vi "20220818_Etalon_with_peak_tracking_for_beam_deviation_working2 .vi"(0 "Session In":T3) -> (4 "vrt. slope":dbl format="%#_9g", 6 "vert intercept":dbl)   [LabVIEW 2021]
uses:
  <vilib>/userDefined/High Color/IMAQdx.ctl
  <vilib>/Analysis/2dsp.llb/Integral Method.ctl
  <vilib>/Analysis/coordinate.llb/2D Cartesian Coordinate Rotation (Array).vi
  <vilib>/Analysis/8numeric.llb/1D Numeric Integration.vi
  <vilib>/Analysis/6fits.llb/Confidence Interval (Linear).vi
  <vilib>/Instr/_visa.llb/VISA Configure Serial Port (Instr).vi
  <vilib>/addons/control/pid/pid.llb/PID (DBL).vi
  <vilib>/Analysis/3filter.llb/Butterworth Filter (DBL).vi
  <vilib>/vision/driver/NI_Vision_Acquisition_Software.lvlib
  <vilib>/Analysis/NI_AALPro.lvlib
  <vilib>/Analysis/NI_AALBase.lvlib
  <vilib>/Analysis/NI_AAL_SigProc.lvlib
  <vilib>/ptbypt/NI_PtbyPt.lvlib
  <resource>/objmgr/imaqdx.rc
  <vilib>/addons/control/pid/NI_PID_pid.lvlib
panel:
  out "second pass wl":dbl format="%#_9g"
  in  "wedge angle (rad)":dbl=0.008737255226 format="%#_13g"
  in  "wedge spacing":dbl=0.8629192 step=1e-06 format="%#_13g"
  in  "pixel size (nm)":dbl=4500.0 format="%#_13g"
  in  "window 2":dbl
  in  "window 1":dbl
  out "Verticle slope (distance between two consecutive fringes)":cluster{dbl[], dbl[]}(graph)
  out "vertical Fringes":dbl[](graph)
  out "Vertical intercept vs real time":cluster{dbl[], dbl[]}(graph)
  out "process variable":dbl
  in  "second peak":i32
  out "Waveform Graph":dbl[](graph)
  out "result 2":dbl format="%0.4f"
  out "Area":dbl
  out "result":dbl format="%0.4f"
  out "First peak pos":dbl
  in  "First peak":i32
  in  "end":dbl format="%.2f"
  in  "index":i32=10
  in  "length":i32=960
  in  "index 2":i32=30
  in  "length 2":i32=700
  out "horzontal intercept":cluster{dbl[], dbl[]}(graph)
  out "horz intercept value":dbl[](array[numeric])
  out "vert wavelength":cluster{dbl[], dbl[]}(graph)
  out "intercept":dbl
  out "x/y":dbl[][](array[numeric])
  out "vert.wl":dbl
  out "d value":dbl format="%#_10e"
  in  "contrast":ext(slide)=0.16666666666666666 scale=0.0..0.3 scale format="%#_12g"
  in  "order 2":i32=2
  in  "order":i32=2
  in  "thor wedge spacing":dbl=4.997771500000001 step=1e-06 format="%#_13g"
  in  "wedge angle of thor wedge":dbl=0.004681980000000043 format="%#_13g"
  in  "horz. fringe width":i32=6 min=3
  out "hor. std dev":dbl format="%0.5f"
  in  "camera property":bool
  in  "saturation":u32(slide) scale=0.0..128.0
  in  "Gain":u32(slide)=49 scale=1.0..256.0
  in  "exposure":ext(slide)=0.49047851562500955 scale=0.000122070313..1.0 scale format="%#_12g"
  out "EnumStrings[]":string[](array[string])
  in  "Numeric":dbl
  out "known wavelength":dbl
  in  "vert width":i32=3 min=3
  out "vert loc":dbl[](array[numeric])
  out "Locations":dbl[](array[numeric])
  out "x > y?":bool
  out "Buffer Number Out":u32
  out "observed wavelength":dbl
  out "horz.intercept":dbl format="%#_8g"
  out "known wl":dbl[](array[numeric])=[591.188, 591.588, 591.988, 592.388, 592.788, 593.188]
  out "obseved wl":dbl[](array[numeric])=[591.1849, 591.5523, 591.984, 592.366, 592.7809, 593.169]
  out "standard deviation":dbl format="%0.5f"
  out "Loop time (ms) 2":u32
  out "Array 3":ext[](array[numeric])
  out "Array 2":dbl[](array[numeric])
  out "Array":dbl[](array[numeric])
  out "count":dbl
  out "horz.slope":dbl format="%#_7g"
  out "?":string
  out "?":string
  out "initial time":u32
  out "initial array vert":ext[](array[numeric])
  out "Y Resolution":i32
  out "X Resolution":i32
  out "initial array horz":ext[](array[numeric])
  out "initila array horz. fringe":ext[](array[numeric])
  in  "Tab Control":enum32{"real time wavelength measurement"}(tab)
  in  "?":T1(tab)
  in  "confidence level vert. fringe":dbl=0.65 format="%.2f"
  in  "threshold vert. fringe":dbl=2.0 min=0.0 max=10.0 step=0.001 format="%0.2f"
  in  "sampling freq. vert. fringe":dbl=2.0 format="%0.2f"
  in  "calibration factor vert. fringe":dbl=1200.0
  in  "confidence level horz. fringe":dbl=0.65 format="%.2f"
  in  "sampling freq. horz. fringe":dbl=1.0 format="%0.2f"
  in  "threshold horz. fringe":dbl=2.0 format="%0.2f"
  in  "calibration factor horz. fringe":dbl=20000.0
  out "RAW Image":T2(plugin-control)
  in  "image depth (bits)":string(combo)="8 bit"
  in  "no. of average":i8=10
  in  "millisecond timer value":u16=100
  in  "sample length":i32=10
  in  "stop":bool
  in  "Calibration":dbl=4.0
  in  "VideoMode":u32=4
  in  "Feedback ON/OFF":bool
  in  "PID gains":T4={"proportional gain (Kc)"=0.01, "integral time (Ti, min)"=0.0, "derivative time (Td, min)"=0.0} {"derivative time (Td, min)" format="%.3f"; "integral time (Ti, min)" format="%.3f"; "proportional gain (Kc)" format="%.3f"}
  out "Output (V)":dbl format="%.2f"
  in  "output range":cluster{"output high":dbl, "output low":dbl}={"output high"=16.0, "output low"=-16.0} {"output low" format="%.2f"; "output high" format="%.2f"}
  out "The raw data (user can select the window \nfor optimum peak for analysis using cursors)":dbl[](graph)
  out "Tracking of the detected peak":dbl[](graph)
  out "Peak detected (peak detected in\n the window selected by user) B":dbl[](graph)
  in  "Threshold for Raw data B":dbl=0.99 format="%0.2f"
  in  "Threshold for\n tracking of detected peak":dbl=0.99 format="%0.2f"
  in  "Window for \ntracking detected peak":i32=40
  out "Error signal":dbl[](graph)
  in  "Window for \npeak detection":i32=60
  out "veertical fringe":dbl[][](graph)
  out "horizontal fringe":dbl[][](graph)
  out "horizontal fringe 2":dbl[][](graph)
  out "initial array vert.  fringe":ext[](array[numeric])
  out "second pass wl 2":dbl format="%#_9g"
  in  "Array length in\n Horiz direction":i32=351
  in  "?":i32=102
  in  "Array length \nin vert direction":i32=65
  in  "Starting position\n in vert direction":i32=50
  in  "Threshold for vert":dbl=0.99 format="%0.2f"
  out "Process Var":dbl
  out "output":dbl format="%.2f"
  in  "setpoint":dbl format="%.2f"
  in  "VISA for power supply 2":refnum<visa-resource-name>
  out "number":i32
  out "read buffer 2":string
  in  "Manual input voltage":dbl format="%.2g"
  in  "Feedback sign":i32=-1 format="%2.0f"
  out "error out 2":errorcluster
  out "error out 3":errorcluster
  out "error out":errorcluster
  # "second pass cal."
  # "To do:\n\n(1)  Include calibration routine\n(3) Statistics: Std error for last N values (N is user selected) 1st pass\n-> statistics for deviation of intercept (in cm-1 or MHz) last N values"
  # "Control parameter"
  # "Fringe selection for analysis"
  # "Starting position in\n Horiz direction"
  # "Set threshold value\n       for peak"
  # "Feedback"
  # "Set window size\n       for peak"
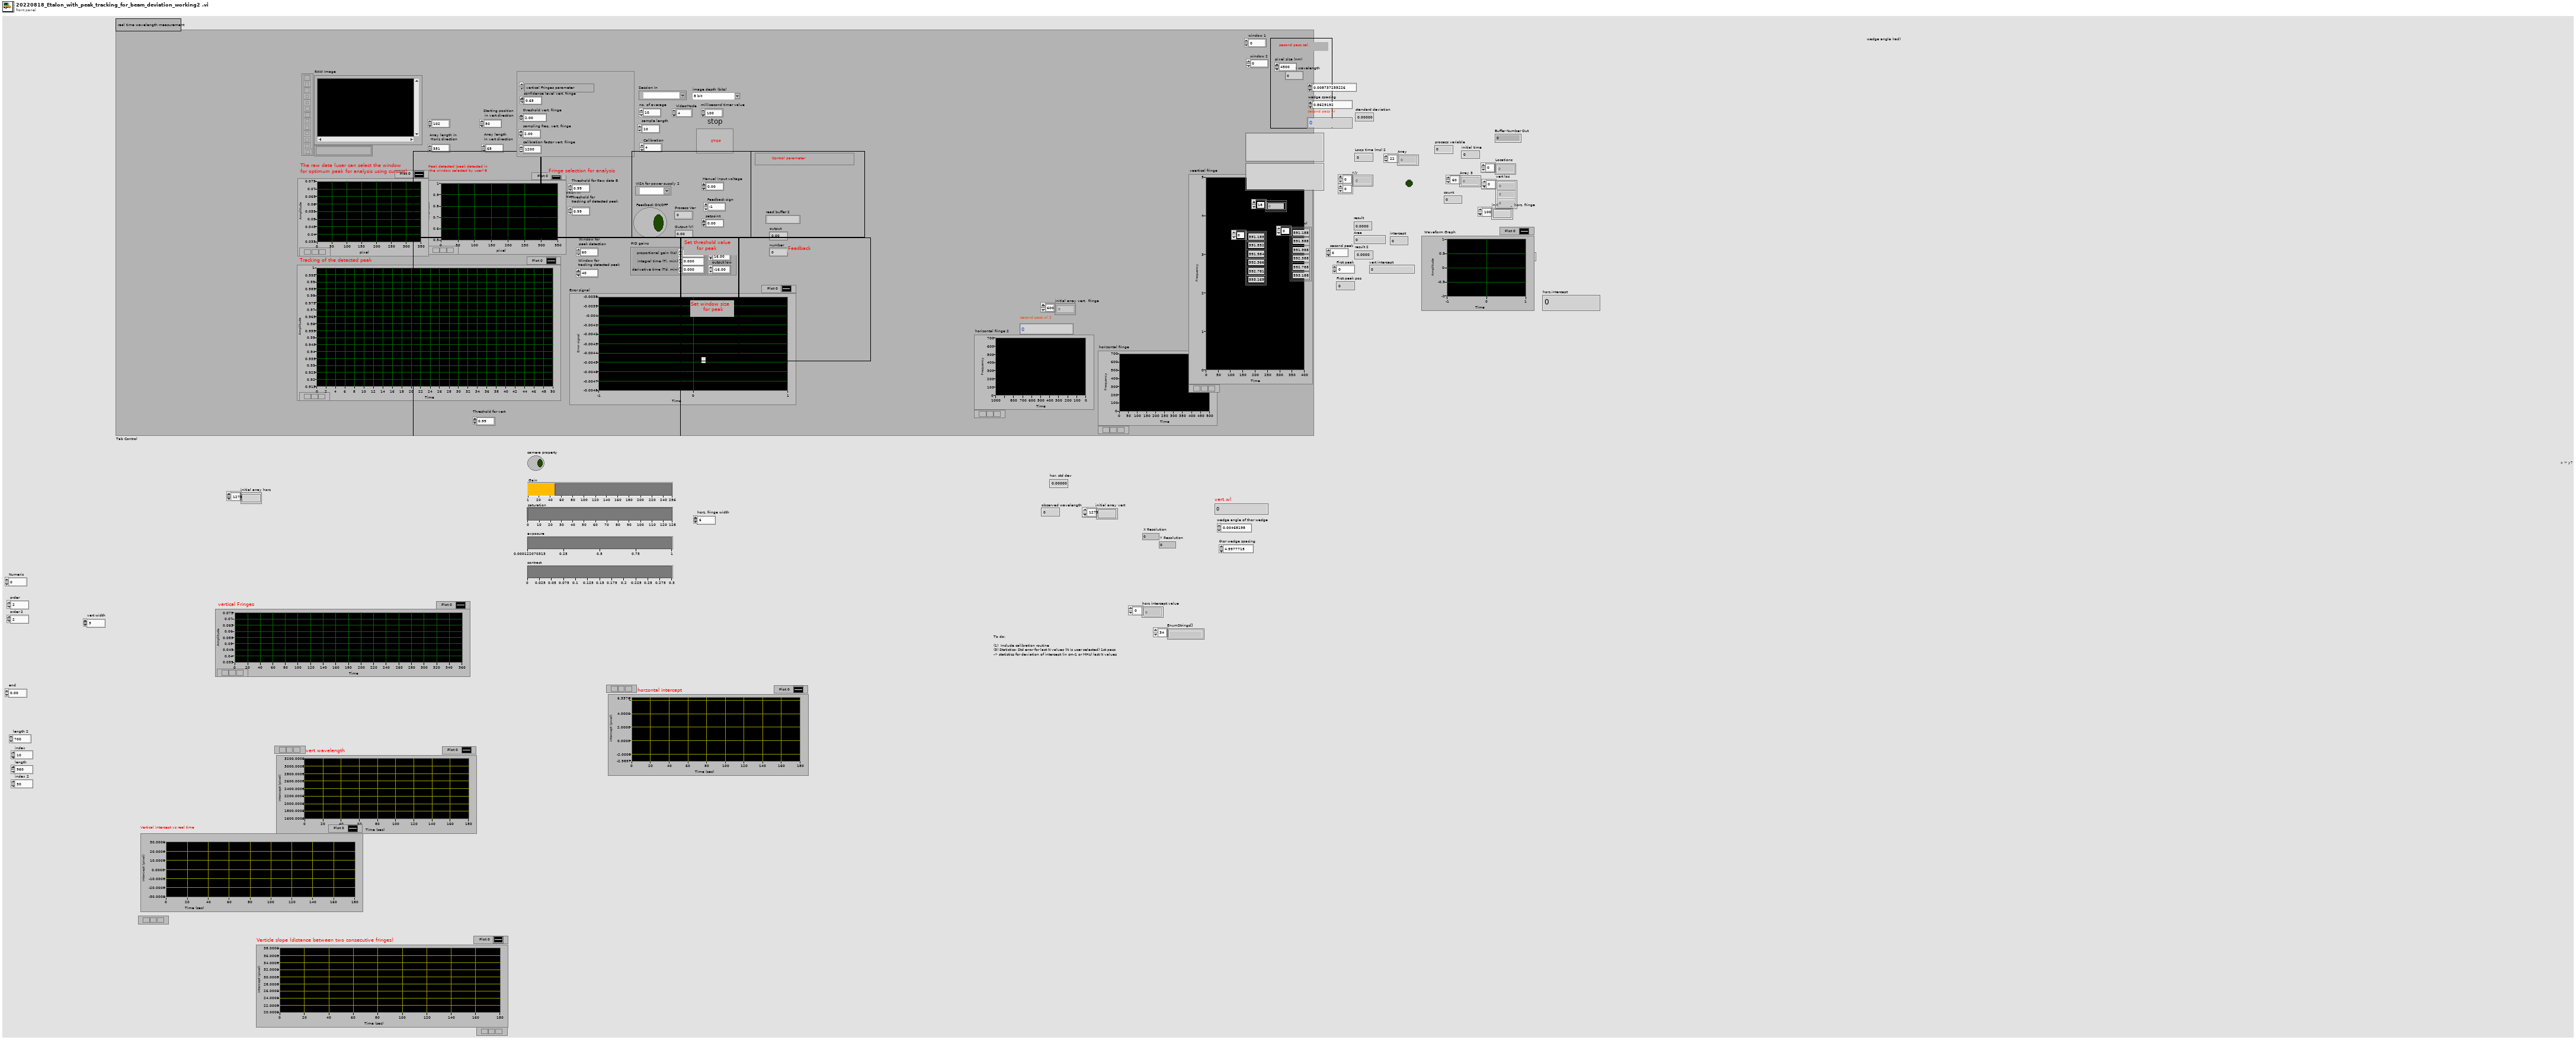
[diagram p1: front panel]
types:
  T1 = enum32{"vertical Fringes parameter", "Horizontal Fringes parameter"}
  T2 = typedef "IMAQ Image.ctl" = refnum<image>
  T3 = typedef "IMAQdx.ctl" = refnum<k21>
  T4 = cluster{"proportional gain (Kc)":dbl, "integral time (Ti, min)":dbl, "derivative time (Td, min)":dbl}
  T5 = typedef "Image Type" = u32
  T6 = typedef "NI_AALPro.lvlib/Integral Method.ctl" = i32
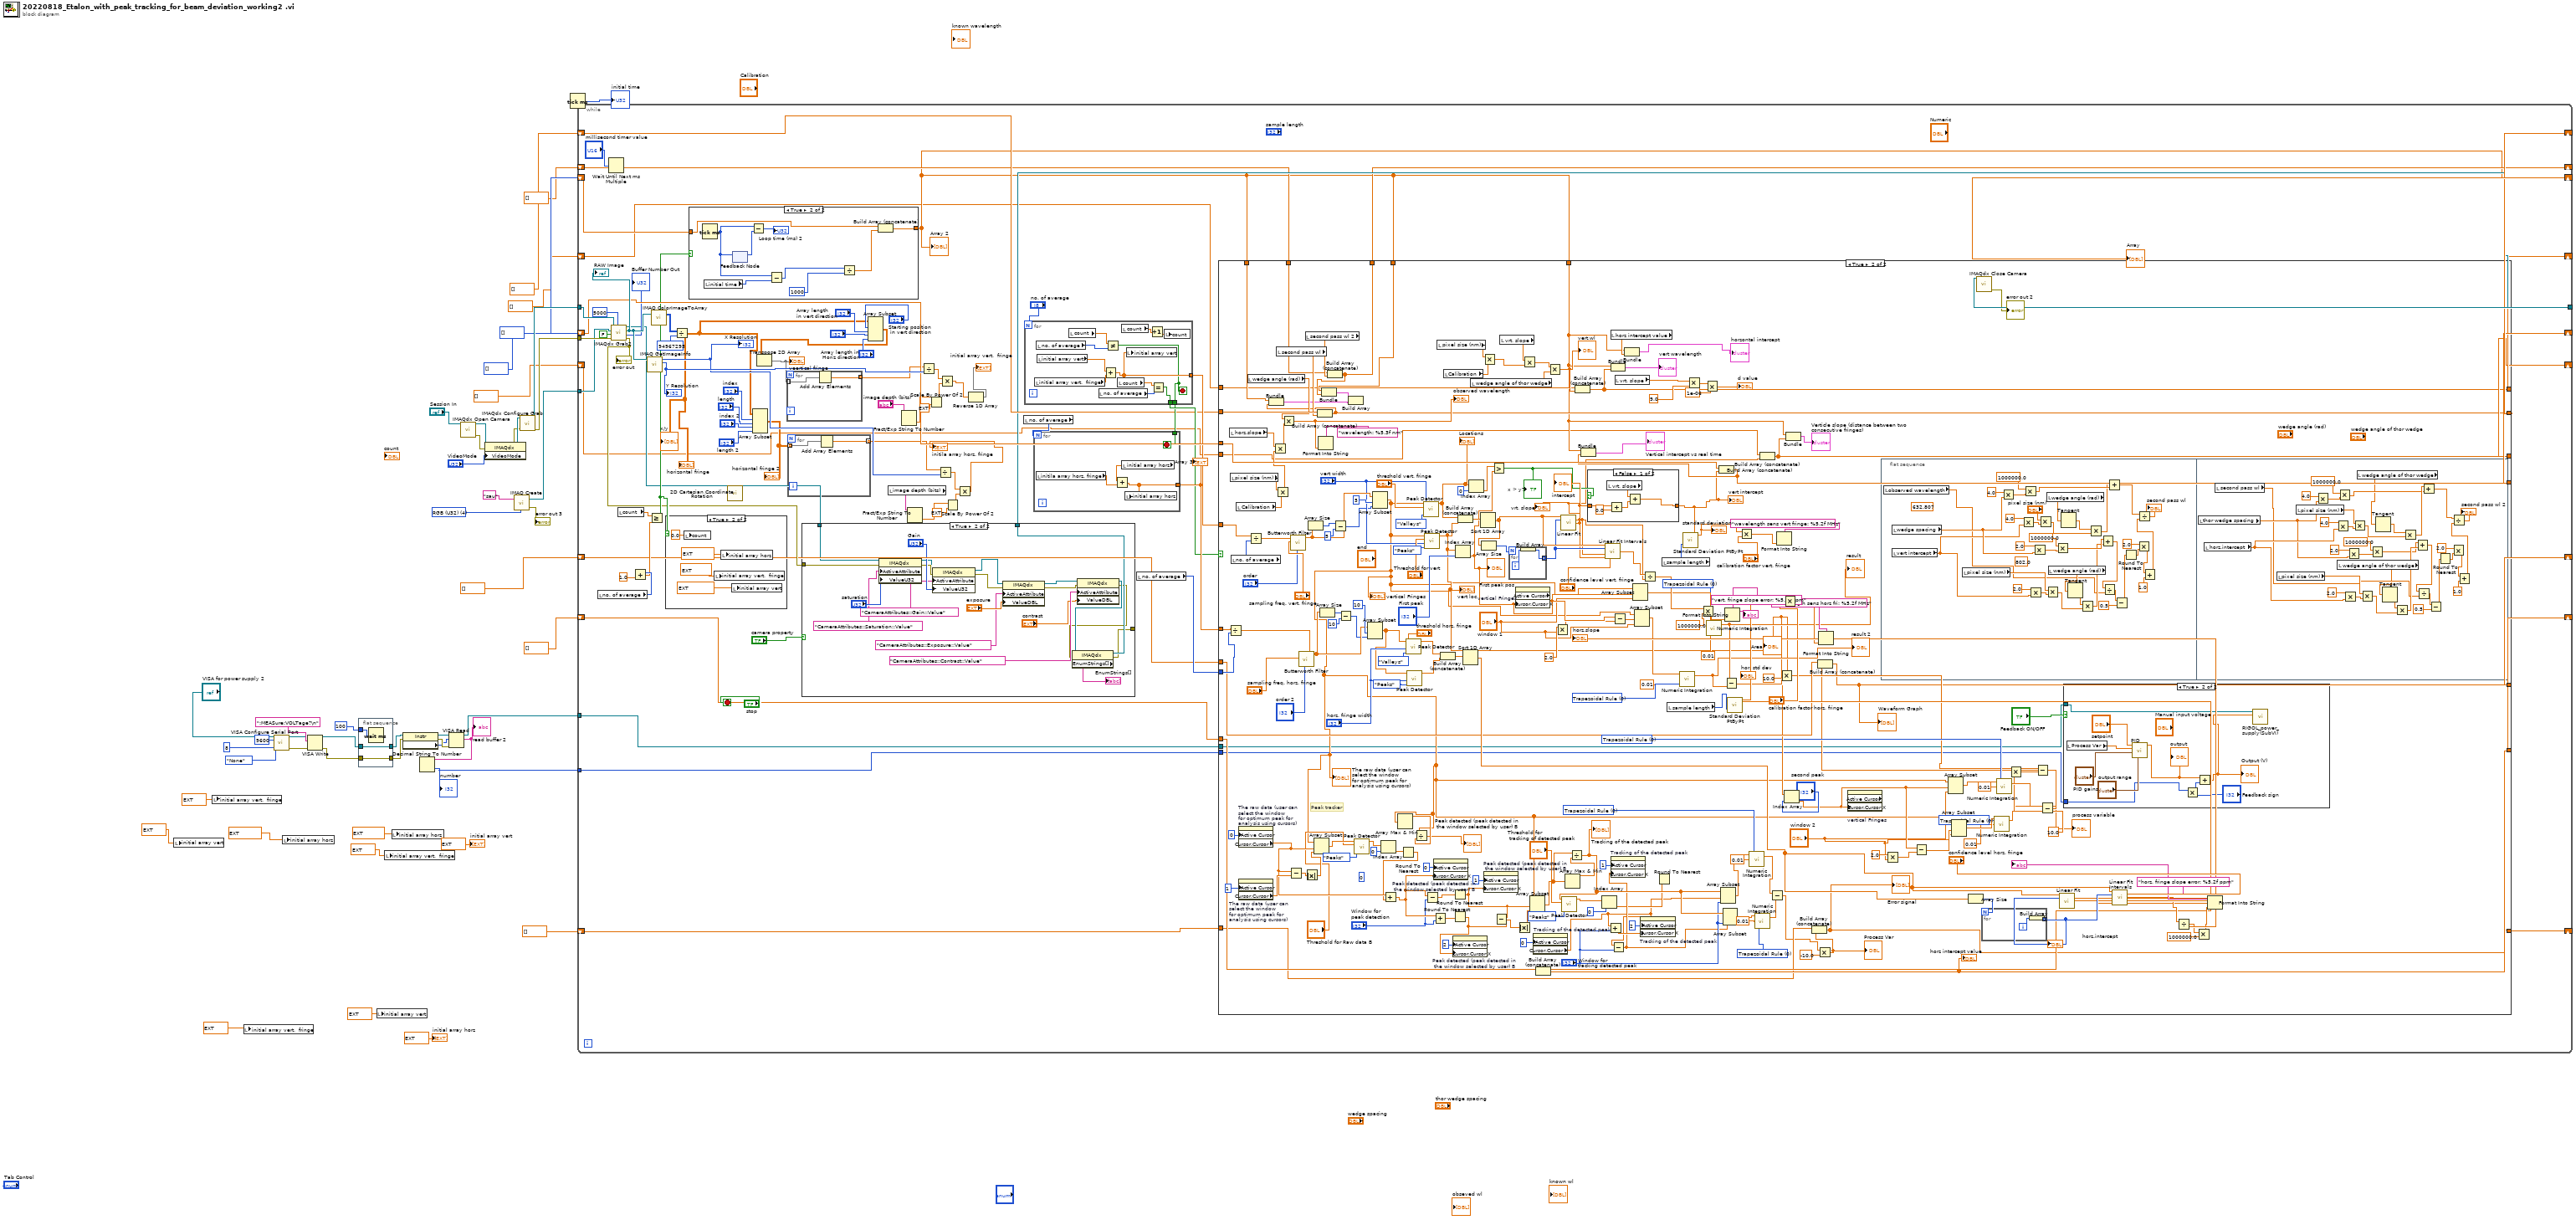
[diagram p0: block diagram]
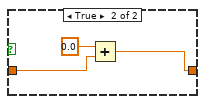
[diagram p7: hidden frame]
diagram:
  w48 = T5 4 items=["Grayscale (U8)", "Grayscale (I16)", "Grayscale (SGL)", "Complex (CSG)", "RGB (U32)", "HSL (U32)", "RGB (U64)", "Grayscale (U16)"] ("Image Type")
  n1 = local write "initial array vert"(ext[] array[1280 elements] ("initial array vert")) -> ()
  n2 = local write "initial array vert.  fringe"(ext[] array[640 elements] ("initial array vert.  fringe")) -> ()
  n3 = local write "initial array vert.  fringe"(ext[] array[1280 elements] ("initial array")) -> ()
  n4 = call-poly "VISA Configure Serial Port"("VISA resource name"="VISA for power supply 2", "baud rate (9600)"=u32 9600, "data bits (8)"=u16 8, "parity (0:none)"=enum16{"None", "Odd", "Even", "Mark", "Space"}."None") -> ("VISA resource name out"=w14:refnum<visa-resource-name>, "error out"=w13:errorcluster)  [unwired: 5 in, 5 out]
  n5 = local write "initial array horz"(ext[] array[1280 elements] ("initial array 2")) -> ()
  n6 = VISA Write(VISA resource name=w14, write buffer=":MEASure:VOLTage?\n" ("Command"), error in (no error)=w13) -> (VISA resource name out=w12:refnum<visa-resource-name>, error out=w11:errorcluster)  [unwired: 1 out]
  n7 = flat-sequence {
    tunnel: w11 -> [w54]
    tunnel: [w54] -> w8
    tunnel: w12 -> [w53]
    tunnel: [w53] -> w9
    tunnel: u32 100 ("delay before read (ms)") -> [w55]
    frame #0 {
      n8 = Wait (ms)(milliseconds to wait=w55) -> ()  [unwired: 1 out]
    }
  }
  n9 = local write "initial array vert"(ext[] array[960 elements] ("initial array vert")) -> ()
  n10 = local write "initial array vert.  fringe"(ext[] array[1280 elements] ("initial array")) -> ()
  n11 = local write "initial array horz"(ext[] array[1280 elements] ("initial array 2")) -> ()
  n12 = property class="Instr"(reference=w9, error in=w8) -> (reference out=w7:refnum<visa-resource-name>, error out=w6:errorcluster, "Serial Settings:Number of Bytes at Serial Port"=w4:u32)
  n13 = VISA Read(VISA resource name=w7, byte count=w4, error in (no error)=w6) -> (VISA resource name out=w2:refnum<visa-resource-name>, read buffer=w5:string)  [unwired: 2 out]
  "read buffer 2" <- w5
  n14 = Decimal String To Number(string=w5) -> (number=w1:i32)  [unwired: 2 in, 1 out]
  "number" <- w1
  n15 = call <vilib>:"IMAQdx Open Camera.vi"("Session In"="Session In") -> ("error out"=w26:errorcluster, "Session Out"=w28:T3)  [unwired: 9 in]
  n16 = property class="IMAQdx"(reference=w28, error in=w26, "VideoMode"="VideoMode") -> (reference out=w27:T3, error out=w25:errorcluster)
  n17 = call "IMAQ Create"("Image Name"="sau", "Image Type"=w48) -> ("New Image"=w46:T2, "error out"=→"error out 3":errorcluster)  [unwired: 3 in]
  n18 = call <vilib>:"IMAQdx Configure Grab.vi"("error in"=w25, "Session In"=w27) -> ("error out"=w45:errorcluster, "Session Out"=w51:T3)  [unwired: 8 in]
  n19 = Tick Count (ms)() -> (millisecond timer value=→"initial time":u32)
  n20 = while {
    tunnel: w45 -> [w129]
    tunnel: w46 -> [w121]
    tunnel: w51 -> [w131]
    tunnel: [w87] -> w42
    shift-right: [w91] -> _
    shift-left: i32[] [] -> [w120]
    shift-right: [w99] -> _
    shift-left: dbl[] [] -> [w93]
    shift-right: [w83] -> w30
    shift-left: u32[] [] -> [w100]
    shift-right: [w84] -> _
    shift-left: dbl[] [] -> [w85]
    shift-right: [w70] -> _
    shift-left: dbl[] [] -> [w69]
    shift-right: [w67] -> _
    shift-left: dbl[] [] -> [w66]
    shift-right: [w62] -> _
    shift-left: dbl[] [] -> [w63]
    shift-right: [w60] -> _
    shift-left: dbl[] [] -> [w61]
    shift-right: [w58] -> _
    shift-left: dbl[] [] -> [w59]
    tunnel: w2 -> [w57]
    tunnel: w1 -> [w56]
    stop <- "stop" stop-if-true
    n21 = local read "no. of average"() -> (w103:i8)
    n22 = Wait Until Next ms Multiple(millisecond multiple="millisecond timer value") -> ()  [unwired: 1 out]
    n23 = call <vilib>:"IMAQdx Grab2.vi"("Timeout (ms)"=5000, "error in"=w129, "Wait for Next Buffer? (Yes)"=FALSE, "Image In"=w121, "Session In"=w131) -> ("error out"=w89:errorcluster, "Buffer Number Out"=→"Buffer Number Out":u32, "Image Out"=w124:T2, "Session Out"=w88:T3)  [unwired: 3 in]
    "error out" <- w89
    "RAW Image" <- w124
    n24 = local read "count"() -> (w105:dbl)
    n25 = Add(x=w103, y=1.0) -> (x+y=w102:dbl)
    n26 = call "IMAQ GetImageInfo"("Image"=w124) -> ("Y Resolution"=w123:i32, "X Resolution"=w122:i32)  [unwired: 3 in, 6 out]
    "Y Resolution" <- w123
    "X Resolution" <- w122
    n27 = Greater Or Equal?(x=w105, y=w102) -> (x >= y?=w101:bool)
    n28 = call "IMAQ ColorImageToArray"("Image"=w124) -> ("Image Pixels (U32)"=w126:u32[][])  [unwired: 3 in, 2 out]
    n29 = case shown="True" w101 {
      frame False {
      }
      frame True {
        n30 = local write "count"(0.0 ("count")) -> ()
        n31 = local write "initial array vert.  fringe"(ext[] array[1280 elements] ("initial array")) -> ()
        n32 = local write "initial array horz"(ext[] array[1280 elements] ("initial array 2")) -> ()
        n33 = local write "initial array vert"(ext[] array[1282 elements] ("initial array vert")) -> ()
      }
    }
    n34 = Divide(x=w126, y=u32 94967295) -> (x/y=w64:dbl[][])
    "horizontal fringe" <- w64
    "x/y" <- w64
    n35 = case shown="True" w101 {
      tunnel: [w155 w158] -> w83
      tunnel: w100 -> [w155 w156]
      frame False {
      }
      frame True {
        n36 = Tick Count (ms)() -> (millisecond timer value=w159:u32)
        n37 = local read "initial time"() -> (w163:u32)
        n38 = feedback #1() -> (w164:u32)  [unwired: 1 in]
        n39 = feedback-in #1(w159) -> ()
        n40 = Subtract(x=w159, y=w164) -> (x-y=→"Loop time (ms) 2":u32)
        n41 = Subtract(x=w159, y=w163) -> (x-y=w160:u32)
        n42 = Divide(x=w160, y=1000) -> (x/y=w157:dbl)
        n43 = Build Array (concatenate)(w156, w157) -> (w158:dbl[])
      }
    }
    "Array 2" <- w83
    n44 = call-poly <vilib>:"2D Cartesian Coordinate Rotation.vi"() -> ()  [unwired: 9 in, 3 out]
    n45 = Array Subset(array=w64, index (row)="index", length (row)="length", index (col)="index 2", length (col)="length 2") -> (w79:dbl[][])
    "horizontal fringe 2" <- w79
    n46 = for {
      tunnel: [w500] -> w115 mode=indexing
      tunnel: w79 -> [w499] mode=indexing
      n47 = Add Array Elements(numeric array=w499) -> (sum=w500:dbl)
    }
    n48 = case shown="True" "camera property" {
      tunnel: w89 -> [w132 w134]
      tunnel: w88 -> [w133 w135]
      tunnel: [w133 w144] -> w87
      tunnel: [w132 w142] -> _
      frame False {
      }
      frame True {
        n49 = property class="IMAQdx"(reference=w135, error in=w134, "ActiveAttribute"="CameraAttributes::Saturation::Value", "ValueU32"="saturation") -> (reference out=w147:T3, error out=w148:errorcluster)
        n50 = property class="IMAQdx"(reference=w147, error in=w148, "ActiveAttribute"="CameraAttributes::Gain::Value", "ValueU32"="Gain") -> (reference out=w152:T3, error out=w151:errorcluster)
        n51 = property class="IMAQdx"(reference=w152, error in=w151, "ActiveAttribute"="CameraAttributes::Exposure::Value", "ValueDBL"="exposure") -> (reference out=w141:T3, error out=w137:errorcluster)
        n52 = property class="IMAQdx"(reference=w141, error in=w137, "ActiveAttribute"="CameraAttributes::Contrast::Value", "ValueDBL"="contrast") -> (reference out=w140:T3, error out=w136:errorcluster)
        n53 = property class="IMAQdx"(reference=w140, error in=w136) -> (reference out=w144:T3, error out=w142:errorcluster, "EnumStrings[]"=→"EnumStrings[]":string[])
      }
    }
    n54 = Array Subset(array=w64, index (row)="Starting position\n in vert direction", length (row)="Array length \nin vert direction", index (col)="?", length (col)="Array length in\n Horiz direction") -> (w74:dbl[][])
    n55 = Transpose 2D Array(2D array=w74) -> (transposed array=w73:dbl[][])
    "veertical fringe" <- w73
    n56 = for {
      tunnel: [w502] -> w119 mode=indexing
      tunnel: w73 -> [w501] mode=indexing
      n57 = Add Array Elements(numeric array=w501) -> (sum=w502:dbl)
    }
    n58 = local read "image depth (bits)"() -> (w94:string)
    n59 = Fract/Exp String To Number(string="image depth (bits)") -> (number=w96:dbl)  [unwired: 3 in, 1 out]
    n60 = Fract/Exp String To Number(string=w94) -> (number=w95:dbl)  [unwired: 3 in, 1 out]
    n61 = Divide(x=w119, y=w123) -> (x/y=w118:dbl[])
    n62 = Scale By Power Of 2(n=w96, x=ext 1.0) -> (x*2^n=w116:ext)
    n63 = Divide(x=w115, y=w122) -> (x/y=w114:dbl[])
    n64 = Multiply(x=w118, y=w116) -> (x*y=w72:ext[])
    n65 = Scale By Power Of 2(n=w95, x=ext 1.0) -> (x*2^n=w112:ext)
    n66 = Multiply(x=w114, y=w112) -> (x*y=→"initila array horz. fringe":ext[])
    n67 = Reverse 1D Array(array=w72) -> (reversed array=→"initial array vert.  fringe":ext[])
    n68 = local read "no. of average"() -> (w108:i8)
    n69 = for {
      N: "no. of average" -> [_]
      tunnel: [w496] -> w109
      tunnel: [w491] -> w107
      tunnel: [w488] -> w106
      stop <- w488 stop-if-true
      n70 = local read "initial array vert.  fringe"() -> (w498:ext[])
      n71 = local read "no. of average"() -> (w489:i8)
      n72 = local read "initial array vert"() -> (w497:ext[])
      n73 = local read "count"() -> (w490:dbl)
      n74 = local read "no. of average"() -> (w495:i8)
      n75 = Add(x=w497, y=w498) -> (x+y=w496:ext[])
      n76 = Not Equal?(x=w490, y=w489) -> (x != y?=w488:bool)
      n77 = local read "count"() -> (w494:dbl)
      n78 = local read "count"() -> (w493:dbl)
      n79 = local write "initial array vert"(w496) -> ()
      n80 = Increment(x=w493) -> (x+1=w492:dbl)
      n81 = Equal?(x=w494, y=w495) -> (x = y?=w491:bool)
      n82 = local write "count"(w492) -> ()
    }
    n83 = for {
      N: w108 -> [_]
      tunnel: [w487] -> w110
      tunnel: w106 -> [w484]
      stop <- w484 stop-if-true
      n84 = local read "initila array horz. fringe"() -> (w485:ext[])
      n85 = local read "initial array horz"() -> (w486:ext[])
      n86 = Add(x=w486, y=w485) -> (x+y=w487:ext[])
      n87 = local write "initial array horz"(w487) -> ()
    }
    "Array 3" <- w110
    n88 = local read "no. of average"() -> (w98:i8)
    n89 = case shown="True" w107 {
      tunnel: [w175 w364] -> w91
      tunnel: w120 -> [w175 w389]
      tunnel: w110 -> [_ w386]
      tunnel: w109 -> [_ w385]
      tunnel: w83 -> [_ w368]
      tunnel: [w176 w308] -> w99
      tunnel: w83 -> [_ w279]
      tunnel: w98 -> [_ w367]
      tunnel: w93 -> [w176 w365]
      tunnel: [w174 w306] -> w84
      tunnel: w85 -> [w174 w309]
      tunnel: w83 -> [_ w307]
      tunnel: [w173 w287] -> w70
      tunnel: w69 -> [w173 w288]
      tunnel: w66 -> [w172 w285]
      tunnel: [w172 w284] -> w67
      tunnel: w63 -> [w171 w278]
      tunnel: [w171 w275] -> w62
      tunnel: w61 -> [w170 w259]
      tunnel: [w170 w235] -> w60
      tunnel: w59 -> [w169 w189]
      tunnel: [w169 w179] -> w58
      tunnel: w57 -> [_ w178]
      tunnel: w56 -> [_ w177]
      frame False {
      }
      frame True {
        w197 = T6 0 items=["Trapezoidal Rule", "Simpson's Rule", "Simpson's 3/8 Rule", "Bode Rule"] ("integration method")
        w200 = T6 0 items=["Trapezoidal Rule", "Simpson's Rule", "Simpson's 3/8 Rule", "Bode Rule"] ("integration method")
        (unwired) u32 0 ("Active Cursor")
        w243 = T6 0 items=["Trapezoidal Rule", "Simpson's Rule", "Simpson's 3/8 Rule", "Bode Rule"] ("integration method")
        w244 = T6 0 items=["Trapezoidal Rule", "Simpson's Rule", "Simpson's 3/8 Rule", "Bode Rule"] ("integration method")
        w264 = T6 0 items=["Trapezoidal Rule", "Simpson's Rule", "Simpson's 3/8 Rule", "Bode Rule"] ("integration method")
        w265 = T6 0 items=["Trapezoidal Rule", "Simpson's Rule", "Simpson's 3/8 Rule", "Bode Rule"] ("integration method")
        # "Peak tracker"
        n90 = Divide(x=w386, y=w367) -> (x/y=w280:ext[])
        n91 = local read "horz.slope"() -> (w335:dbl)
        n92 = local read "pixel size (nm)"() -> (w328:dbl)
        n93 = local read "no. of average"() -> (w387:i8)
        n94 = local read "Calibration"() -> (w330:dbl)
        n95 = property on="The raw data (user can select the window \nfor optimum peak for analysis using cursors)" class="WFGraph (strict)"("Active Cursor"=u32 0) -> ("Cursor.Cursor X"=w214:dbl)  [unwired: 2 in, 2 out]
        n96 = property on="The raw data (user can select the window \nfor optimum peak for analysis using cursors)" class="WFGraph (strict)"("Active Cursor"=u32 1) -> ("Cursor.Cursor X"=w215:dbl)  [unwired: 2 in, 2 out]
        n97 = local read "wedge angle (rad)"() -> (w331:dbl)
        n98 = Divide(x=w385, y=w387) -> (x/y=w388:ext[])
        n99 = Multiply(x=w328, y=w330) -> (x*y=w329:dbl)
        n100 = Multiply(x=w335, y=w329) -> (x*y=w334:dbl)
        n101 = local read "second pass wl"() -> (w333:dbl)
        n102 = Multiply(x=w331, y=w334) -> (x*y=w332:dbl)
        "observed wavelength" <- w332
        n103 = Subtract(x=w214, y=w215) -> (x-y=w234:dbl)
        n104 = call-poly <vilib>:"Butterworth Filter.vi"("order"="order", "sampling freq: fs"="sampling freq. vert. fringe", "X"=w388) -> ("Filtered X"=w338:dbl[])  [unwired: 5 in, 1 out]
        n105 = call-poly <vilib>:"Butterworth Filter.vi"("order"="order 2", "sampling freq: fs"="sampling freq. horz. fringe", "X"=w280) -> ("Filtered X"=w320:dbl[])  [unwired: 5 in, 1 out]
        n106 = Absolute Value(x=w234) -> (abs(x)=w233:dbl)
        n107 = local read "second pass wl 2"() -> (w310:dbl)
        n108 = Array Size(array=w338) -> (size(s)=w316:i32)
        n109 = Build Array (concatenate)(w365, w333) -> (w308:dbl[])
        n110 = Bundle(w368, w308) -> (w304:cluster{dbl[], dbl[]})  [unwired: 1 in]
        n111 = Format Into String(format string="wavelength: %5.3f nm", w332) -> ()  [unwired: 2 in, 2 out]
        n112 = Array Size(array=w320) -> (size(s)=w319:i32)
        n113 = Build Array (concatenate)(w309, w310) -> (w306:dbl[])
        n114 = Bundle(w307, w306) -> (w305:cluster{dbl[], dbl[]})  [unwired: 1 in]
        n115 = Subtract(x=w316, y=5) -> (x-y=w314:i32)
        n116 = Subtract(x=w319, y=10) -> (x-y=w318:i32)
        n117 = Build Array(w305, w304) -> ()  [unwired: 1 out]
        n118 = Array Subset(array=w320, index=10, length=w318) -> (w181:dbl[])
        n119 = Array Subset(array=w338, index=5, length=w314) -> (w180:dbl[])
        "vertical Fringes" <- w180
        "The raw data (user can select the window \nfor optimum peak for analysis using cursors)" <- w180
        n120 = Array Subset(array=w180, index=w214, length=w233) -> (w232:dbl[])
        n121 = call <vilib>:"Peak Detector.vi"("peaks/valleys"=enum32{"Peaks", "Valleys"}."Peaks", "threshold"="Threshold for Raw data B", "X"=w232) -> ("Locations"=w230:dbl[])  [unwired: 4 in, 4 out]
        n122 = Index Array(array=w230, index=0) -> (element=w206:dbl)
        n123 = Array Max & Min(array=w180) -> (max value=w209:dbl)  [unwired: 3 out]
        n124 = Round To Nearest(number=w206) -> (nearest integer value=w205:dbl)
        n125 = Add(x=w214, y=w205) -> (x+y=w227:dbl)
        n126 = call <vilib>:"Peak Detector.vi"("peaks/valleys"=enum32{"Peaks", "Valleys"}."Valleys", "width"="horz. fringe width", "threshold"="threshold horz. fringe", "X"=w181) -> ("Locations"=w359:dbl[])  [unwired: 3 in, 4 out]
        n127 = call <vilib>:"Peak Detector.vi"("peaks/valleys"=enum32{"Peaks", "Valleys"}."Peaks", "width"="horz. fringe width", "X"=w181) -> ("Locations"=w358:dbl[])  [unwired: 4 in, 4 out]
        n128 = Divide(x=w180, y=w209) -> (x/y=→"Peak detected (peak detected in\n the window selected by user) B":dbl[])
        n129 = call <vilib>:"Peak Detector.vi"("peaks/valleys"=enum32{"Peaks", "Valleys"}."Valleys", "width"="vert width", "threshold"="threshold vert. fringe", "X"=w180) -> ("Locations"=w345:dbl[])  [unwired: 3 in, 4 out]
        "Locations" <- w345
        n130 = call <vilib>:"Peak Detector.vi"("peaks/valleys"=enum32{"Peaks", "Valleys"}."Peaks", "width"="vert width", "threshold"="Threshold for vert", "X"=w180) -> ("Locations"=w255:dbl[])  [unwired: 3 in, 4 out]
        "vert loc" <- w255
        n131 = Subtract(x=w227, y="Window for \npeak detection") -> (x-y=w223:dbl)
        n132 = Add(x=w227, y="Window for \npeak detection") -> (x+y=w222:dbl)
        n133 = property on="Peak detected (peak detected in\n the window selected by user) B" class="WFGraph (strict)"("Active Cursor"=u32 0, "Cursor.Cursor X"=w227) -> ()  [unwired: 2 in, 2 out]
        n134 = local read "pixel size (nm)"() -> (w296:dbl)
        n135 = Build Array (concatenate)(w359, w358) -> (w357:dbl[])
        n136 = local read "Calibration"() -> (w295:dbl)
        n137 = Round To Nearest(number=w223) -> (nearest integer value=w221:dbl)
        n138 = Round To Nearest(number=w222) -> (nearest integer value=w220:dbl)
        n139 = property on="Peak detected (peak detected in\n the window selected by user) B" class="WFGraph (strict)"("Active Cursor"=u32 2, "Cursor.Cursor X"=w220) -> ()  [unwired: 2 in, 2 out]
        n140 = Index Array(array=w255, index="First peak") -> (element=w272:dbl)
        "First peak pos" <- w272
        n141 = Build Array (concatenate)(w345, w255) -> (w381:dbl[])
        n142 = Sort 1D Array(array=w357) -> (sorted array=w354:dbl[])
        n143 = Index Array(array=w345, index=0) -> (element=w343:dbl)
        n144 = local read "wedge angle of thor wedge"() -> (w291:dbl)
        n145 = Sort 1D Array(array=w381) -> (sorted array=w379:dbl[])
        n146 = Array Size(array=w379) -> (size(s)=w380:i32)
        n147 = Multiply(x=w296, y=w295) -> (x*y=w293:dbl)
        n148 = property on="Peak detected (peak detected in\n the window selected by user) B" class="WFGraph (strict)"("Active Cursor"=u32 1, "Cursor.Cursor X"=w221) -> ()  [unwired: 2 in, 2 out]
        n149 = Greater?(x=w343, y=w272) -> (0:w342:bool)
        "x > y?" <- w342
        n150 = Subtract(x=w221, y=w220) -> (x-y=w213:dbl)
        n151 = local read "vrt. slope"() -> (w294:dbl)
        n152 = for {
          N: w380 -> [_]
          tunnel: [w483] -> w378 mode=concatenating
          i -> [w482]
          n153 = Build Array(w482) -> (w483:i32[])
        }
        n154 = property on="vertical Fringes" class="WFGraph (strict)" props=["Active Cursor", "Cursor", "Cursor X"]("Cursor.Cursor X"=w272) -> ()  [unwired: 2 in, 3 out]
        n155 = Absolute Value(x=w213) -> (abs(x)=w212:dbl)
        n156 = Multiply(x=w294, y=w293) -> (x*y=w292:dbl)
        n157 = Array Subset(array=w180, index=w221, length=w212) -> (w211:dbl[])
        n158 = property on="Tracking of the detected peak" class="WFGraph (strict)"("Active Cursor"=u32 0) -> ("Cursor.Cursor X"=w185:dbl)  [unwired: 2 in, 2 out]
        n159 = Multiply(x=w292, y=w291) -> (x*y=w286:dbl)
        "vert.wl" <- w286
        n160 = Multiply(x=2.0, y="window 1") -> (x*y=w271:dbl)
        n161 = call <vilib>:"Linear Fit.vi"("Y"=w379, "X"=w378) -> ("slope"=w277:dbl, "intercept"=w346:dbl)  [unwired: 9 in, 3 out]
        "vrt. slope" <- w277
        "intercept" <- w346
        n162 = Array Max & Min(array=w211) -> (max value=w210:dbl)  [unwired: 3 out]
        n163 = Divide(x=w211, y=w210) -> (x/y=w203:dbl[])
        "Tracking of the detected peak" <- w203
        n164 = call <vilib>:"Peak Detector.vi"("peaks/valleys"=enum32{"Peaks", "Valleys"}."Peaks", "threshold"="Threshold for\n tracking of detected peak", "X"=w203) -> ("Locations"=w188:dbl[])  [unwired: 4 in, 4 out]
        n165 = Build Array (concatenate)(w285, w286) -> (w284:dbl[])
        n166 = case shown="False" w342 {
          tunnel: w346 -> [w402 w407]
          tunnel: [w404 w406] -> w290
          frame False {
            n167 = local read "vrt. slope"() -> (w403:dbl)
            n168 = Add(x=w402, y=0.0) -> (x+y=w401:dbl)
            n169 = Add(x=w403, y=w401) -> (x+y=w404:dbl)
          }
          frame True {
            n170 = Add(x=0.0, y=w407) -> (x+y=w406:dbl)
          }
        }
        "vert intercept" <- w290
        n171 = Index Array(array=w188, index=0) -> (element=w186:dbl)
        n172 = call-poly <vilib>:"Linear Fit Intervals.vi"("Y"=w379, "confidence level"="confidence level vert. fringe", "X"=w378, "slope"=w277, "intercept"=w346) -> ("delta slope"=w374:dbl)  [unwired: 6 in, 4 out]
        n173 = Add(x=w185, y="Window for \ntracking detected peak") -> (x+y=w191:dbl)
        n174 = local read "horz intercept value"() -> (w282:dbl[])
        n175 = Bundle(w279, w284) -> (→"vert wavelength":cluster{dbl[], dbl[]})  [unwired: 1 in]
        n176 = Subtract(x=w185, y="Window for \ntracking detected peak") -> (x-y=w190:dbl)
        n177 = property on="Tracking of the detected peak" class="WFGraph (strict)"("Active Cursor"=u32 1, "Cursor.Cursor X"=w190) -> ()  [unwired: 2 in, 2 out]
        n178 = Subtract(x=w272, y=w271) -> (x-y=w270:dbl)
        n179 = local read "vrt. slope"() -> (w303:dbl)
        n180 = Bundle(w279, "horz intercept value"=w282) -> (→"horzontal intercept":cluster{dbl[], "horz intercept value":dbl[]})  [unwired: 1 in]
        n181 = Array Subset(array=w180, index=w272, length="window 1") -> (w267:dbl[])
        n182 = Array Subset(array=w180, index=w270, length="window 1") -> (w266:dbl[])
        n183 = property on="Tracking of the detected peak" class="WFGraph (strict)"("Active Cursor"=u32 2, "Cursor.Cursor X"=w191) -> ()  [unwired: 2 in, 2 out]
        n184 = Divide(x=w374, y=w277) -> (x/y=w373:dbl)
        n185 = Round To Nearest(number=w186) -> ()  [unwired: 1 out]
        n186 = local read "sample length"() -> (w311:i32)
        n187 = local read "sample length"() -> (w325:i32)
        n188 = call-poly <vilib>:"Numeric Integration.vi"("integration method"=w264, "dt"=0.01 ("dt 3"), "Input Array"=w266) -> ("result"=w260:dbl)  [unwired: 1 out]
        "result 2" <- w260
        n189 = call <vilib>:"Standard Deviation PtByPt.vi"("x"=w290, "sample length"=w311) -> ("standard deviation"=w369:dbl)  [unwired: 1 in, 2 out]
        "standard deviation" <- w369
        n190 = Multiply(x=w303, y=9.0) -> (x*y=w301:dbl)
        n191 = Multiply(x=w373, y=1000000.0) -> (x*y=w372:dbl)
        n192 = Multiply(x=w301, y=1e-06) -> (x*y=→"d value":dbl)
        n193 = call-poly <vilib>:"Numeric Integration.vi"("integration method"=w265, "dt"=0.01 ("dt 2"), "Input Array"=w267) -> ("result"=w261:dbl)  [unwired: 1 out]
        "result" <- w261
        n194 = Build Array (concatenate)(w389, w290) -> (w364:dbl[])
        n195 = Bundle(w279, w364) -> (→"Vertical intercept vs real time":cluster{dbl[], dbl[]})  [unwired: 1 in]
        n196 = Array Subset(array=w203, index=w185, length="Window for \ntracking detected peak") -> (w202:dbl[])
        n197 = Array Subset(array=w203, index=w190, length="Window for \ntracking detected peak") -> (w199:dbl[])
        n198 = Subtract(x=w261, y=w260) -> (x-y=w257:dbl)
        "Area" <- w257
        n199 = Format Into String(format string="vert. fringe slope error: %5.2f ppm", w372) -> (resulting string=→"?":string)  [unwired: 2 in, 1 out]
        n200 = Multiply(x=w369, y="calibration factor vert. fringe") -> (x*y=w370:dbl)
        n201 = call-poly <vilib>:"Numeric Integration.vi"("integration method"=w200, "dt"=0.01, "Input Array"=w202) -> ("result"=w196:dbl)  [unwired: 1 out]
        n202 = call-poly <vilib>:"Numeric Integration.vi"("integration method"=w197, "dt"=0.01, "Input Array"=w199) -> ("result"=w195:dbl)  [unwired: 1 out]
        n203 = Build Array (concatenate)(w278, w277) -> (w275:dbl[])
        n204 = Subtract(x=w196, y=w195) -> (x-y=w183:dbl)
        n205 = Format Into String(format string="wavelength sens vert fringe: %5.2f MHz", w370) -> ()  [unwired: 2 in, 2 out]
        n206 = Multiply(x=w257, y=10.0) -> (x*y=w238:dbl)
        n207 = Index Array(array=w255, index="second peak") -> (element=w254:dbl)
        n208 = Bundle(w279, w275) -> (→"Verticle slope (distance between two consecutive fringes)":cluster{dbl[], dbl[]})  [unwired: 1 in]
        n209 = Multiply(x=w183, y=-10.0) -> (x*y=w182:dbl)
        "Process Var" <- w182
        n210 = Build Array (concatenate)(w189, w182) -> (w179:dbl[])
        "Error signal" <- w179
        n211 = property on="vertical Fringes" class="WFGraph (strict)" props=["Active Cursor", "Cursor", "Cursor X"]("Cursor.Cursor X"=w254) -> ()  [unwired: 2 in, 3 out]
        n212 = flat-sequence {
          frame #0 {
            (unwired) 632.807 ("x")
            (unwired) 802.0
            n213 = local read "observed wavelength"() -> (w410:dbl)
            n214 = local read "wedge spacing"() -> (w414:dbl)
            n215 = local read "vert intercept"() -> (w413:dbl)
            n216 = local read "pixel size (nm)"() -> (w416:dbl)
            n217 = Multiply(x=4.0, y=w414) -> (x*y=w443:dbl)
            n218 = Multiply(x=4.0, y=w413) -> (x*y=w439:dbl)
            n219 = Multiply(x=1000000.0, y=w443) -> (x*y=w442:dbl)
            n220 = Multiply(x=2.0, y=w413) -> (x*y=w428:dbl)
            n221 = Multiply(x=2.0, y=w414) -> (x*y=w433:dbl)
            n222 = Multiply(x="pixel size (nm)", y=w439) -> (x*y=w437:dbl)
            n223 = Multiply(x=w416, y=w428) -> (x*y=w425:dbl)
            n224 = local read "wedge angle (rad)"() -> (w415:dbl)
            n225 = local read "wedge angle (rad)"() -> (w411:dbl)
            n226 = Multiply(x=1000000.0, y=w433) -> (x*y=w429:dbl)
            n227 = Tangent(1:w415) -> (0:w438:dbl)
            n228 = Tangent(1:w411) -> (0:w426:dbl)
            n229 = Multiply(x=w426, y=w425) -> (x*y=w421:dbl)
            n230 = Multiply(x=w438, y=w437) -> (x*y=w436:dbl)
            n231 = Add(x=w429, y=w421) -> (x+y=w420:dbl)
            n232 = Divide(x=w420, y=w410) -> (x/y=w424:dbl)
            n233 = Add(x=w436, y=w442) -> (x+y=w431:dbl)
            n234 = Subtract(x=w424, y=0.5) -> (x-y=w422:dbl)
            n235 = Round To Nearest(number=w422) -> (nearest integer value=w418:dbl)
            n236 = Multiply(x=2.0, y=w418) -> (x*y=w417:dbl)
            n237 = Add(x=w417, y=1.0 ("x")) -> (x+y=w430:dbl)
            n238 = Divide(x=w431, y=w430) -> (x/y=→"second pass wl":dbl)
          }
          frame #1 {
            n239 = local read "thor wedge spacing"() -> (w479:dbl)
            n240 = local read "horz.intercept"() -> (w480:dbl)
            n241 = local read "second pass wl"() -> (w450:dbl)
            n242 = local read "pixel size (nm)"() -> (w478:dbl)
            n243 = local read "pixel size (nm)"() -> (w451:dbl)
            n244 = Multiply(x=4.0, y=w479) -> (x*y=w453:dbl)
            n245 = Multiply(x=4.0, y=w480) -> (x*y=w456:dbl)
            n246 = Multiply(x=1000000.0, y=w453) -> (x*y=w454:dbl)
            n247 = local read "wedge angle of thor wedge"() -> (w449:dbl)
            n248 = Multiply(x=2.0, y=w480) -> (x*y=w466:dbl)
            n249 = Multiply(x=2.0, y=w479) -> (x*y=w461:dbl)
            n250 = Multiply(x=w451, y=w456) -> (x*y=w458:dbl)
            n251 = local read "wedge angle of thor wedge"() -> (w448:dbl)
            n252 = Multiply(x=w478, y=w466) -> (x*y=w469:dbl)
            n253 = Multiply(x=1000000.0, y=w461) -> (x*y=w465:dbl)
            n254 = Tangent(1:w448) -> (0:w457:dbl)
            n255 = Tangent(1:w449) -> (0:w468:dbl)
            n256 = Multiply(x=w468, y=w469) -> (x*y=w473:dbl)
            n257 = Multiply(x=w457, y=w458) -> (x*y=w459:dbl)
            n258 = Add(x=w465, y=w473) -> (x+y=w474:dbl)
            n259 = Divide(x=w474, y=w450) -> (x/y=w470:dbl)
            n260 = Add(x=w459, y=w454) -> (x+y=w463:dbl)
            n261 = Subtract(x=w470, y=0.5) -> (x-y=w472:dbl)
            n262 = Round To Nearest(number=w472) -> (nearest integer value=w476:dbl)
            n263 = Multiply(x=2.0, y=w476) -> (x*y=w477:dbl)
            n264 = Add(x=w477, y=1.0 ("x")) -> (x+y=w464:dbl)
            n265 = Divide(x=w463, y=w464) -> (x/y=→"second pass wl 2":dbl)
          }
        }
        n266 = Multiply(x=2.0, y="window 2") -> (x*y=w251:dbl)
        n267 = Subtract(x=w254, y=w251) -> (x-y=w253:dbl)
        n268 = Array Subset(array=w180, index=w254, length="window 2") -> (w248:dbl[])
        n269 = Array Subset(array=w180, index=w253, length="window 2") -> (w247:dbl[])
        n270 = Array Size(array=w354) -> (size(s)=w356:i32)
        n271 = for {
          N: w356 -> [_]
          tunnel: [w409] -> w355 mode=concatenating
          i -> [w408]
          n272 = Build Array(w408) -> (w409:i32[])
        }
        n273 = call-poly <vilib>:"Numeric Integration.vi"("integration method"=w243, "dt"=0.01, "Input Array"=w247) -> ("result"=w241:dbl)  [unwired: 1 out]
        n274 = call-poly <vilib>:"Numeric Integration.vi"("integration method"=w244, "dt"=0.01, "Input Array"=w248) -> ("result"=w242:dbl)  [unwired: 1 out]
        n275 = Subtract(x=w242, y=w241) -> (x-y=w239:dbl)
        n276 = Multiply(x=w239, y=10.0) -> (x*y=w237:dbl)
        n277 = Subtract(x=w238, y=w237) -> (x-y=w236:dbl)
        "process variable" <- w236
        n278 = Build Array (concatenate)(w259, w236) -> (w235:dbl[])
        "Waveform Graph" <- w235
        n279 = call <vilib>:"Linear Fit.vi"("Y"=w354, "X"=w355) -> ("slope"=w350:dbl, "intercept"=w289:dbl)  [unwired: 9 in, 3 out]
        "horz.slope" <- w350
        "horz.intercept" <- w289
        n280 = Build Array (concatenate)(w288, w289) -> (w287:dbl[])
        "horz intercept value" <- w287
        n281 = call <vilib>:"Standard Deviation PtByPt.vi"("x"=w289, "sample length"=w325) -> ("standard deviation"=w327:dbl)  [unwired: 1 in, 2 out]
        "hor. std dev" <- w327
        n282 = Multiply(x=w327, y="calibration factor horz. fringe") -> (x*y=w326:dbl)
        n283 = Format Into String(format string="wavelength sens horz fri: %5.2f MHz", w326) -> ()  [unwired: 2 in, 2 out]
        n284 = case shown="True" "Feedback ON/OFF" {
          tunnel: w178 -> [_ w394]
          tunnel: w177 -> [_ w393]
          frame False {
          }
          frame True {
            n285 = local read "Process Var"() -> (w397:dbl)
            n286 = call-poly <vilib>:"PID.vi"("output range"="output range", "PID gains"="PID gains", "process variable"=w397, "setpoint"="setpoint") -> ("output"=w396:dbl)  [unwired: 6 in, 1 out]
            "output" <- w396
            n287 = Multiply(x=w393, y="Feedback sign") -> (x*y=w391:i32)
            n288 = Add(x=w396, y=w391) -> (x+y=w390:dbl)
            "Output (V)" <- w390
            n289 = call "RIGOL_power_supply(SubVI).vi"("voltage_in 3"=w390, "VISA Refnum in"=w394) -> ()  [unwired: 8 in, 2 out]
          }
        }
        n290 = call-poly <vilib>:"Linear Fit Intervals.vi"("Y"=w354, "confidence level"="confidence level horz. fringe", "X"=w355, "slope"=w350, "intercept"=w289) -> ("delta slope"=w323:dbl)  [unwired: 6 in, 4 out]
        n291 = Divide(x=w323, y=w350) -> (x/y=w348:dbl)
        n292 = Multiply(x=w348, y=1000000.0) -> (x*y=w347:dbl)
        n293 = Format Into String(format string="horz. fringe slope error: %5.2f ppm", w347) -> (resulting string=→"?":string)  [unwired: 2 in, 1 out]
      }
    }
  }
  "Array" <- w30
  n294 = call <vilib>:"IMAQdx Close Camera.vi"("Session In"=w42) -> ("error out"=→"error out 2":errorcluster)  [unwired: 10 in]
  "initial array horz" <- ext[] array[960 elements] ("initial array horz")
  "initial array vert" <- ext[] array[1280 elements] ("initial array vert")
